vi "Test Reset.vi"(8 "error in (no error)":errorcluster, 11 "Test Case In":refnum<class "Debug Latest Message Test.lvclass">) -> (0 "error out":errorcluster, 3 "Test Case Out":refnum<class "Debug Latest Message Test.lvclass">)   [LabVIEW 2020, in "Debug Latest Message Test.lvclass"]
uses:
  Debug Latest Message Test.lvclass
  Debug Latest Message Test.lvclass/Debug Latest Message Test.ctl
  01074fa8-ee8a-411d-bc8b-fc92c4f90959.vi
  source/Debug Latest Message/Debug Latest Message.lvclass
  source/Debug Data/Raw Debug Data.ctl
  source/Debug Data/Debug Data.lvclass
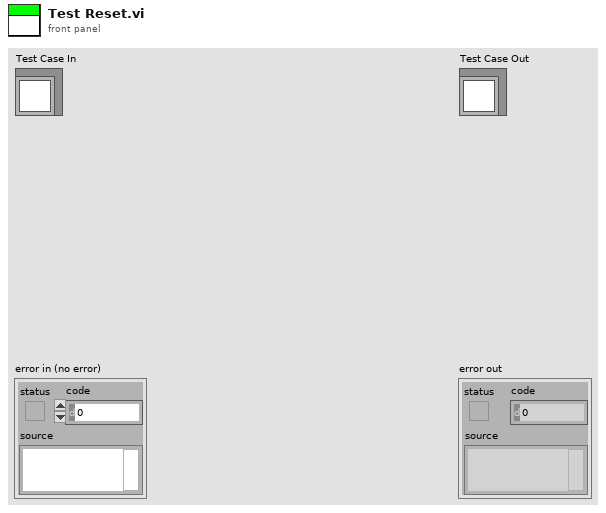
[diagram p1: front panel]
types:
  T1 = typedef "Debug Data.lvclass/Raw Debug Data.ctl" = cluster{"Action":string, "Call Chain":string, "Process":string, "Message":string, "Message Data":variant, "Time":dbl}
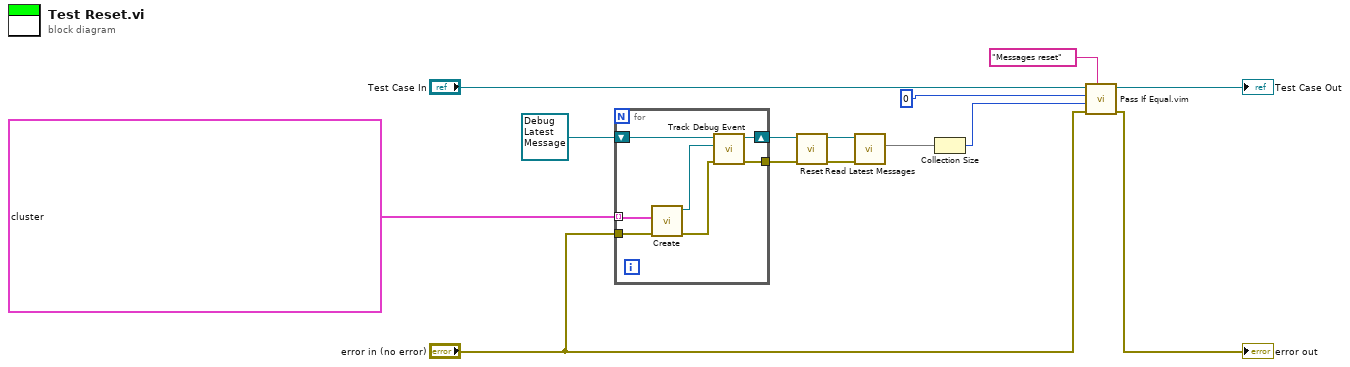
[diagram p0: block diagram]
diagram:
  n1 = for {
    tunnel: [w20] -> w11
    shift-right: [w21] -> w4
    shift-left: refnum<class "Debug Latest Message.lvclass"> refnum ("Debug Latest Message in") -> [w19]
    tunnel: T1[] [{"Action"="Send", "Call Chain"="Test.vi:123456", "Process"="Process 1", "Message"="Init", "Message Data"=variant, "Time"=0.0}, {"Action"="Receive", "Call Chain"="TF.lvlib:Process.lvclass:Handle Messages.vi:1960001", "Process"="Process 1", "Message"="Init", "Message Data"=variant, "Time"=0.0}, {"Action"="Send", "Call Chain"="Test.vi", "Process"="Process 1", "Message"="Start", "Message Data"=variant, "Time"=0.0}] ("Debug Data Cluster") -> [w18] mode=indexing
    tunnel: "error in (no error)" -> [w17]
    n2 = call "Create.vi"("error in (no error)"=w17, "Debug Data Cluster"=w18) -> ("error out"=w16:errorcluster, "Debug Data out"=w15:refnum<class "Debug Data.lvclass">)  [unwired: 8 in]
    n3 = call "Track Debug Event.vi"("error in (no error)"=w16, "Debug Data.lvclass"=w15, "Debug Latest Message In"=w19) -> ("error out"=w20:errorcluster, "Debug Latest Message Out"=w21:refnum<class "Debug Latest Message.lvclass">)  [unwired: 7 in]
  }
  n4 = call "Reset.vi"("error in (no error)"=w11, "Debug Latest Message in"=w4) -> ("error out"=w5:errorcluster, "Debug Latest Message out"=w3:refnum<class "Debug Latest Message.lvclass">)  [unwired: 8 in]
  n5 = call "Read Latest Messages.vi"("error in (no error)"=w5, "Debug Latest Message in"=w3) -> ("Latest Messages"=w2:map{string, refnum<class "Debug Data.lvclass">})  [unwired: 7 in, 2 out]
  n6 = Collection Size(1:w2) -> (0:w7:i32)
  n7 = call "Pass If Equal.vim"("Description"="Messages reset", "error in (no error)"="error in (no error)", "Actual"=w7, "Expected"=0 ("size"), "LUnit Test Case In"="Test Case In") -> ("error out"=→"error out":errorcluster, "LUnit Test Case Out"=→"Test Case Out":refnum<class "Debug Latest Message Test.lvclass">)  [unwired: 5 in]
